vi "Scale_Graph_Y (SubVI).vi"(6 "AktYSkl":u8, 9 "Array":dbl[](array[numeric]), 10 "Faktor":dbl, 11 "XYGraph (Eingang)":refnum<vi>) -> ()   [LabVIEW 2014]
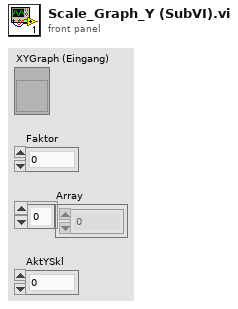
[diagram p1: front panel]
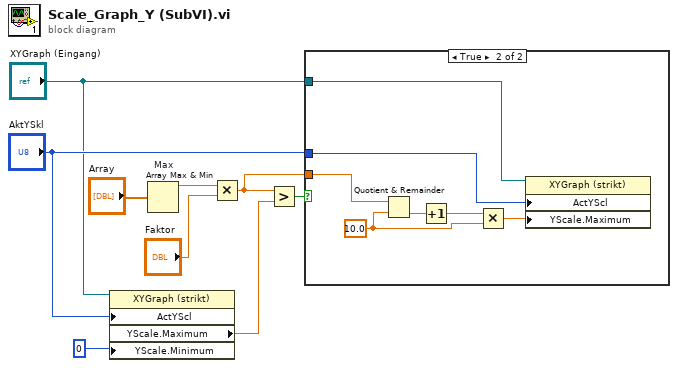
[diagram p0: block diagram]
diagram:
  n1 = property on="Eigenschaftsknoten" class="XYGraph (strikt)"(reference="XYGraph (Eingang)", "ActYScl"="AktYSkl", "YScale.Minimum"=0) -> ("YScale.Maximum"=w6:dbl)  [unwired: 1 in, 2 out]
  n2 = Array Max & Min "Max"(array="Array") -> (max value=w7:dbl)  [unwired: 3 out]
  n3 = Multiply(x=w7, y="Faktor") -> (x*y=w4:dbl)
  n4 = Greater?(x=w4, y=w6) -> (0:w5:bool)
  n5 = case shown="True" w5 {
    tunnel: w4 -> [_ w13]
    tunnel: "AktYSkl" -> [_ w11]
    tunnel: "XYGraph (Eingang)" -> [_ w10]
    frame False {
    }
    frame True {
      w14 = 10.0
      n6 = Quotient & Remainder(x=w13, y=w14) -> (floor(x/y)=w15:dbl)  [unwired: 1 out]
      n7 = Increment(x=w15) -> (x+1=w16:dbl)
      n8 = Multiply(x=w16, y=w14) -> (x*y=w12:dbl)
      n9 = property on="Eigenschaftsknoten" class="XYGraph (strikt)"(reference=w10, "ActYScl"=w11, "YScale.Maximum"=w12) -> ()  [unwired: 1 in, 2 out]
    }
  }
